vi "m1m3_getEvent_PowerWarning.vi"(8 "error in (no error)":errorcluster, 11 "logevent_PowerWarning_Ctl":T1) -> (0 "error out":errorcluster, 2 "function return":i32, 3 "logevent_PowerWarning_Ctl out":T1)   [LabVIEW 2016, in "SALLV_m1m3.lvlib"]
doc: "int m1m3_shm_getEvent_PowerWarningLV(m1m3_logevent_PowerWarningLV *logevent_PowerWarning_Ctl );"
uses:
  SALLV_m1m3.lvlib
  DataTypes/logevent_PowerWarning.ctl
  SALLV_m1m3.so
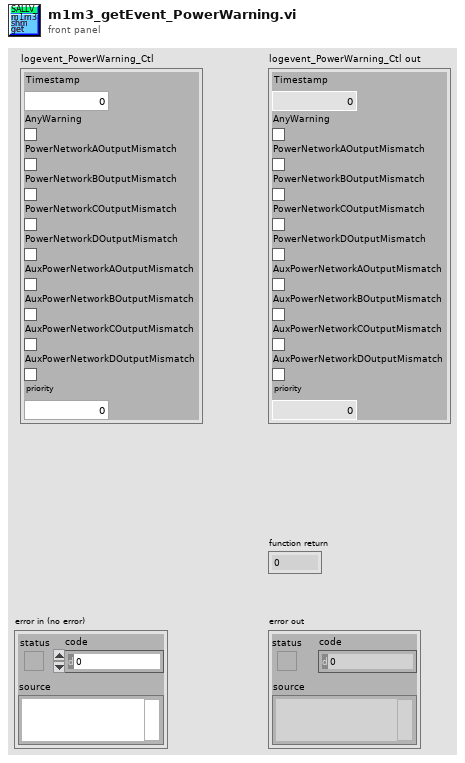
[diagram p1: front panel]
types:
  T1 = typedef "SALLV_m1m3.lvlib/logevent_PowerWarning.ctl" = cluster{"Timestamp":dbl, "AnyWarning":bool, "PowerNetworkAOutputMismatch":bool, "PowerNetworkBOutputMismatch":bool, "PowerNetworkCOutputMismatch":bool, "PowerNetworkDOutputMismatch":bool, "AuxPowerNetworkAOutputMismatch":bool, "AuxPowerNetworkBOutputMismatch":bool, "AuxPowerNetworkCOutputMismatch":bool, "AuxPowerNetworkDOutputMismatch":bool, "priority":i32}
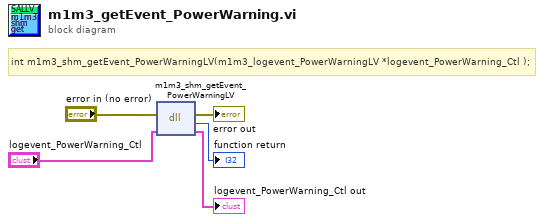
[diagram p0: block diagram]
diagram:
  # "int m1m3_shm_getEvent_PowerWarningLV(m1m3_logevent_PowerWarningLV *logevent_PowerWarning_Ctl );"
  n1 = dll-call lib="opt/CODE/SALLV_m1m3/SALLV_m1m3.*" fn="m1m3_shm_getEvent_PowerWarningLV"(error in="error in (no error)", "logevent_PowerWarning_Ctl"="logevent_PowerWarning_Ctl") -> (error out=→"error out":errorcluster, →"function return":i32, "logevent_PowerWarning_Ctl"=→"logevent_PowerWarning_Ctl out":T1)  [unwired: 2 in, 1 out]
